vi "DISP_WIND_TRAC_STAT.vi"(0 "VISA IN":refnum<visa-resource-name>, 1 "Trace":i32=1, 2 "ON | OFF":bool, 5 "error in":errorcluster, 7 "Window":i32=1) -> (14 "VISA Out":refnum<visa-resource-name>, 19 "error out":errorcluster)   [LabVIEW 2018, in "PNA-X.lvlib"]
doc: "DISPlay:WINDow<wnum>:TRACe<tnum>[:STATe] <ON | OFF> \n(Read-Write) Turns the display of the specified trace in the specified window ON or OFF. When OFF, \nthe measurement behind the trace is still active. \nParameters \n<wnum> Any existing window number. If unspecified, value is set to 1. \n<tnum> Any existing trace number; if unspecified, value is set to 1 \n<ON | OFF> ON (or 1) - turns the trace ON. \nOFF (or 0) - turns the trace OFF. \nExamples DISP:WIND:TRAC ON \ndisplay:window2:trace2:state off \nQuery Syntax DISPlay:WIND<wnum>:TRACe<tnum>[:STATe]? \nReturn Type Boolean (1 = ON, 0 = OFF) \nDefault ON"
uses:
  PNA-X.lvlib
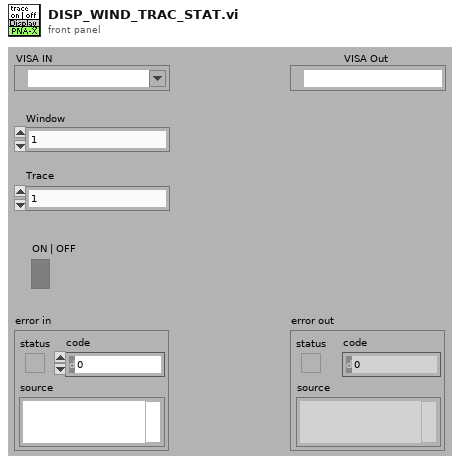
[diagram p1: front panel]
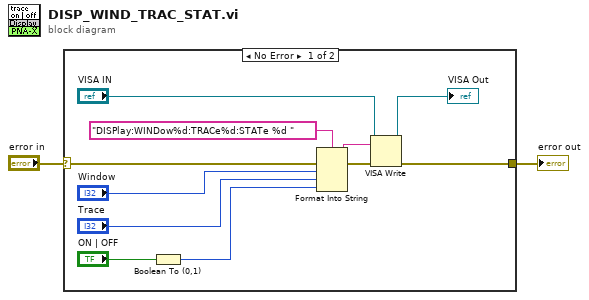
[diagram p0: block diagram]
diagram:
  n1 = case shown="No Error" "error in" {
    selector: "error in" -> [w13 w14]
    tunnel: [w8 w14] -> w1
    frame No Error {
      n2 = Boolean To (0,1)(Boolean="ON | OFF") -> (0, 1=w3:i16)
      n3 = Format Into String(format string="DISPlay:WINDow%d:TRACe%d:STATe %d " ("Cmdline"), error in=w13, "Window", "Trace", w3) -> (resulting string=w11:string, error out=w12:errorcluster)  [unwired: 1 in]
      n4 = VISA Write(VISA resource name="VISA IN", write buffer=w11, error in (no error)=w12) -> (VISA resource name out=→"VISA Out":refnum<visa-resource-name>, error out=w8:errorcluster)  [unwired: 1 out]
    }
    frame Error {
    }
  }
  "error out" <- w1
